vi "LLA_SubVI_string.vi"(11 "read buffer":string) -> (1 "Alt":dbl, 2 "Long":dbl, 3 "Lat":dbl)   [LabVIEW 2016]
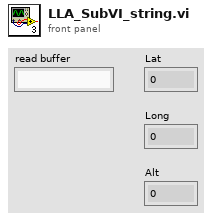
[diagram p1: front panel]
types:
  T1 = enum16{"big-endian, network order", "native, host order", "little-endian"}
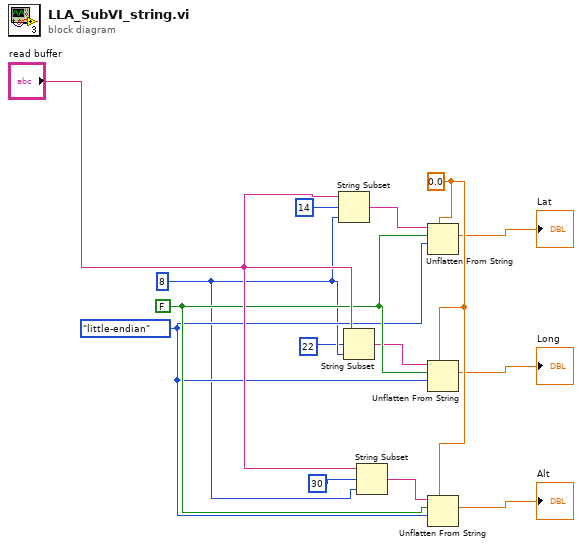
[diagram p0: block diagram]
diagram:
  w13 = 0.0
  w12 = FALSE ("data includes array or string size? (T)")
  w11 = T1."little-endian" ("byte order (0:big-endian, network order)")
  w10 = 8
  n1 = String Subset(string="read buffer", offset (0)=14, length (rest)=w10) -> (substring=w7:string)
  n2 = String Subset(string="read buffer", offset (0)=22, length (rest)=w10) -> (substring=w4:string)
  n3 = String Subset(string="read buffer", offset (0)=30, length (rest)=w10) -> (substring=w1:string)
  n4 = Unflatten From String(type=w13, binary string=w7, data includes array or string size? (T)=w12, byte order (0:big-endian, network order)=w11) -> (value=→"Lat":dbl)  [unwired: 1 in, 2 out]
  n5 = Unflatten From String(type=w13, binary string=w4, data includes array or string size? (T)=w12, byte order (0:big-endian, network order)=w11) -> (value=→"Long":dbl)  [unwired: 1 in, 2 out]
  n6 = Unflatten From String(type=w13, binary string=w1, data includes array or string size? (T)=w12, byte order (0:big-endian, network order)=w11) -> (value=→"Alt":dbl)  [unwired: 1 in, 2 out]
